vi "Status 0 Read.vi"(4 "error in (no error)":errorcluster, 6 "Container State":T2, 7 "Display State In":T1={"State 1"={"BG"=0, "FG"=0}, "State 0"={"BG"=0, "FG"=0}, "State 2"={"BG"=0, "FG"=0}, "State 3"={"BG"=0, "FG"=0}, "Shortcut Menu"=enum."Do left-click popup"}) -> (0 "error out":errorcluster, 2 "Value":cluster{"BG":u32, "FG":u32}, 3 "Display State Out":T1={"State 1"={"BG"=0, "FG"=0}, "State 0"={"BG"=0, "FG"=0}, "State 2"={"BG"=0, "FG"=0}, "State 3"={"BG"=0, "FG"=0}, "Shortcut Menu"=enum."Do left-click popup"})   [LabVIEW 2011, in "Led.xctl"]
uses:
  Led.xctl
  <vilib>/_xctls/Container State.ctl
  State.ctl
  <vilib>/_xctls/XControlSupport.lvlib
panel:
  # "Replace the Value Indicator below with an Indicator of desired type.\nDo not remove this Indicator or the others from the connector pane. \nDo not change the connector pane pattern.\nThe Value Indicator should always be the second terminal from top on the output side in the connector pane."
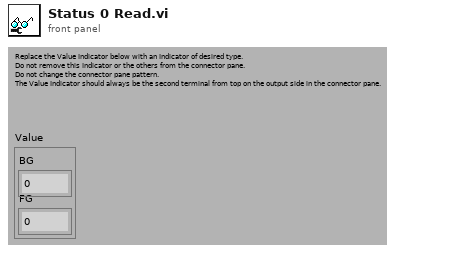
[diagram p1: front panel]
types:
  T1 = typedef "Led.xctl/State.ctl" = cluster{"State 1":cluster{"BG":u32, "FG":u32}, "State 0":cluster{"BG":u32, "FG":u32}, "State 2":cluster{"BG":u32, "FG":u32}, "State 3":cluster{"BG":u32, "FG":u32}, "Shortcut Menu":enum16{"Treat normally", "Do left-click popup"}}
  T2 = typedef "XControlSupport.lvlib/Container State.ctl" = cluster{"Indicator?":bool, "Run Mode?":bool, " Refnum":refnum<vi>}
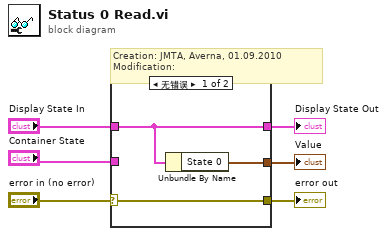
[diagram p0: block diagram]
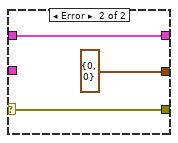
[diagram p2: hidden frame]
diagram:
  # "Creation: JMTA, Averna, 01.09.2010 \nModification:"
  n1 = case shown="无错误" "error in (no error)" {
    selector: "error in (no error)" -> [w9 w11]
    tunnel: "Display State In" -> [w8 w12]
    tunnel: [w9 w11] -> w4
    tunnel: [w8 w12] -> w3
    tunnel: "Container State" -> [_ _]
    tunnel: [w7 cluster{"BG":u32, "FG":u32} {"BG"=0, "FG"=0} ("Value")] -> w1
    frame No Error {
      n2 = Unbundle By Name(w8) -> ("State 0"=w7:cluster{"BG":u32, "FG":u32})
    }
    frame Error {
    }
  }
  "error out" <- w4
  "Display State Out" <- w3
  "Value" <- w1
